vi "Get Sift Proxy Params.vi"(8 "error in (no error)":errorcluster, 11 "Sift Client in":refnum<class "Sift Client.lvclass">) -> (0 "error out":errorcluster, 1 "Log Path":path, 2 "Sift Proxy Address":string, 3 "Sift Client out":refnum<class "Sift Client.lvclass">)   [LabVIEW 2024, in "Sift Client.lvlib" / "Sift Client.lvclass"]
uses:
  Sift Client.lvclass
  Sift Client.lvclass/Sift Client.ctl
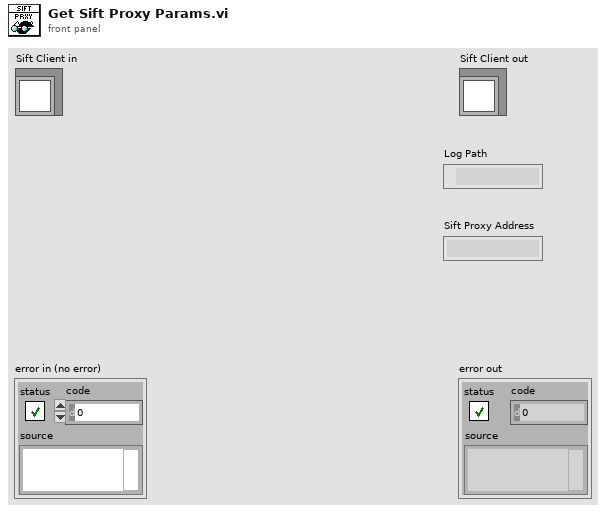
[diagram p1: front panel]
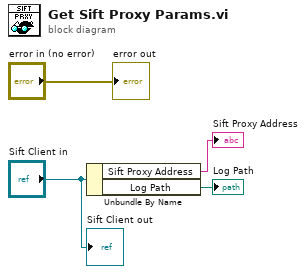
[diagram p0: block diagram]
diagram:
  n1 = Unbundle By Name("Sift Client in") -> ("Sift Proxy Address"=→"Sift Proxy Address":string, "Log Path"=→"Log Path":path)
  "error out" <- "error in (no error)"
  "Sift Client out" <- "Sift Client in"
